vi "Read clientCertificates.vi"(8 "error in (no error)":errorcluster, 11 "dotNET SSL Client Socket in":refnum<class "dotNET SSL Client Socket.lvclass">) -> (0 "error out":errorcluster, 2 "clientCertificates":refnum<k24>, 3 "dotNET SSL Client Socket out":refnum<class "dotNET SSL Client Socket.lvclass">)   [LabVIEW 2013, in "dotNET SSL Socket.lvlib" / "dotNET SSL Client Socket.lvclass"]
uses:
  dotNET SSL Client Socket.lvclass
  dotNET SSL Client Socket.lvclass/dotNET SSL Client Socket.ctl
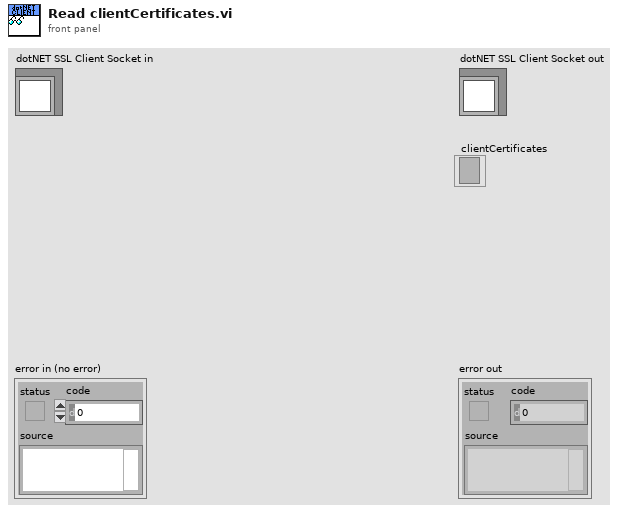
[diagram p1: front panel]
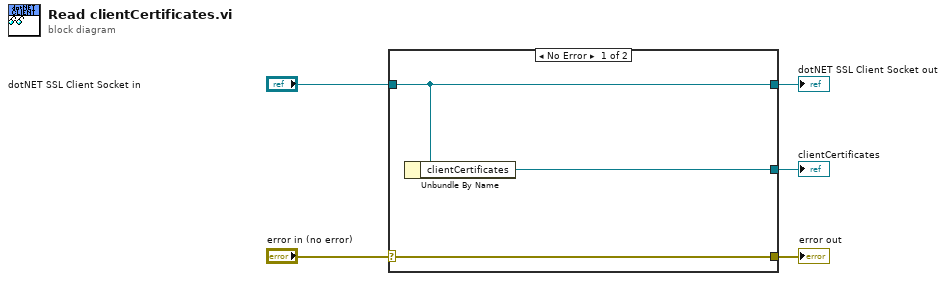
[diagram p0: block diagram]
diagram:
  n1 = case shown="No Error" "error in (no error)" {
    selector: "error in (no error)" -> [w8 w9]
    tunnel: [w8 w9] -> w4
    tunnel: [w7 w10] -> w2
    tunnel: "dotNET SSL Client Socket in" -> [w7 w10]
    tunnel: [w6 _] -> w1
    frame No Error {
      n2 = Unbundle By Name(w7) -> ("clientCertificates"=w6:refnum<k24>)
    }
    frame Error {
    }
  }
  "error out" <- w4
  "dotNET SSL Client Socket out" <- w2
  "clientCertificates" <- w1
